vi "AudioStreamer.Create Graph.vi"(7 "waveforms":waveform(sgl)[](array[waveform])) -> (8 "plot":waveform(sgl)[](array[waveform]))   [LabVIEW 2020]
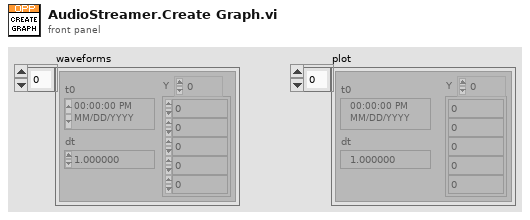
[diagram p1: front panel]
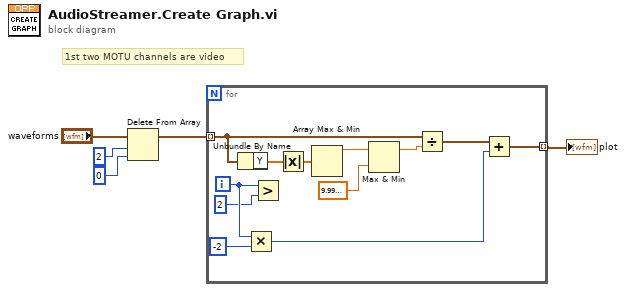
[diagram p0: block diagram]
diagram:
  # "1st two MOTU channels are video"
  n1 = Delete From Array(array="waveforms", length=2, index=0) -> (array with subset deleted=w2:waveform(sgl)[])  [unwired: 1 out]
  n2 = for {
    tunnel: w2 -> [w11] mode=indexing
    tunnel: [w17] -> w1 mode=indexing
    i -> [w14]
    n3 = Unbundle By Name(w11) -> ("Y"=w10:sgl[])
    n4 = Multiply(x=w14, y=-2 ("x")) -> (x*y=w16:i32)
    n5 = Greater?(x=w14, y=2) -> ()  [unwired: 1 out]
    n6 = Absolute Value(x=w10) -> (abs(x)=w9:sgl[])
    n7 = Array Max & Min(array=w9) -> (max value=w8:sgl)  [unwired: 3 out]
    n8 = Max & Min(x=w8, y=sgl 1e-06) -> (max(x,y)=w6:sgl)  [unwired: 1 out]
    n9 = Divide(x=w11, y=w6) -> (x/y=w12:waveform(sgl))
    n10 = Add(x=w12, y=w16) -> (x+y=w17:waveform(sgl))
  }
  "plot" <- w1
